vi "wrapper_get_stopThread.vi"(0 "HGF_ThreadWorker in":refnum<class "HGF_ThreadWorker.lvclass">, 5 "error in (no error)":errorcluster) -> (14 "HGF_ThreadWorker out":refnum<class "HGF_ThreadWorker.lvclass">, 16 "stopThread":bool, 19 "error out":errorcluster)   [LabVIEW 2014, in "HGF_BaseClasses.lvlib" / "HGF_ThreadWorker.lvclass"]
doc: "protected dynamic dispatch wrapper VI to allow childClass access"
uses:
  HGF_ThreadWorker.lvclass
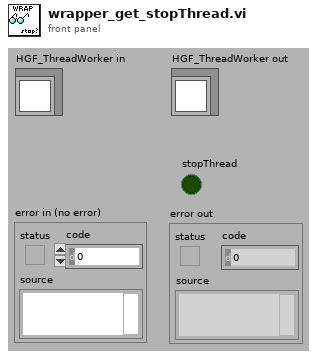
[diagram p1: front panel]
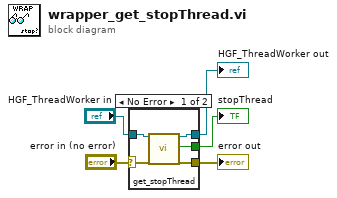
[diagram p0: block diagram]
diagram:
  n1 = case shown="No Error" "error in (no error)" {
    selector: "error in (no error)" -> [w7 w12]
    tunnel: [w6 w12] -> w4
    tunnel: [w9 w11] -> w2
    tunnel: "HGF_ThreadWorker in" -> [w10 w11]
    tunnel: [w8 _] -> w1
    frame No Error {
      n2 = call "get_stopThread.vi"("HGF_ThreadWorker"=w10, "error in (no error)"=w7) -> ("dup HGF_ThreadWorker"=w9:refnum<class "HGF_ThreadWorker.lvclass">, "stopThread"=w8:bool, "error out"=w6:errorcluster)  [unwired: 15 in]
    }
    frame Error {
    }
  }
  "error out" <- w4
  "HGF_ThreadWorker out" <- w2
  "stopThread" <- w1
